vi "String to Parameter Type.vi"(0 "String in":string) -> (4 "Message Name":string, 6 "Parameters":T1[](array[typedef]), 8 "Parameter-1553":T1)   [LabVIEW 2011, in "AIT 1553 Custom Device.lvlib"]
uses:
  Controls/1553 Param.ctl
  AIT 1553 Custom Device.lvlib
panel:
  out "array":string[][](array[string])
  # "Message: Gun_One\nData_01,8,0,8,1.0000,0.0000,0\nMessage: Gun_Two\nData_02,8,0,8,1.0000,0.0000,0\nMessage: Get_It\nData_00,1,0,8,1.0000,0.0000,0"
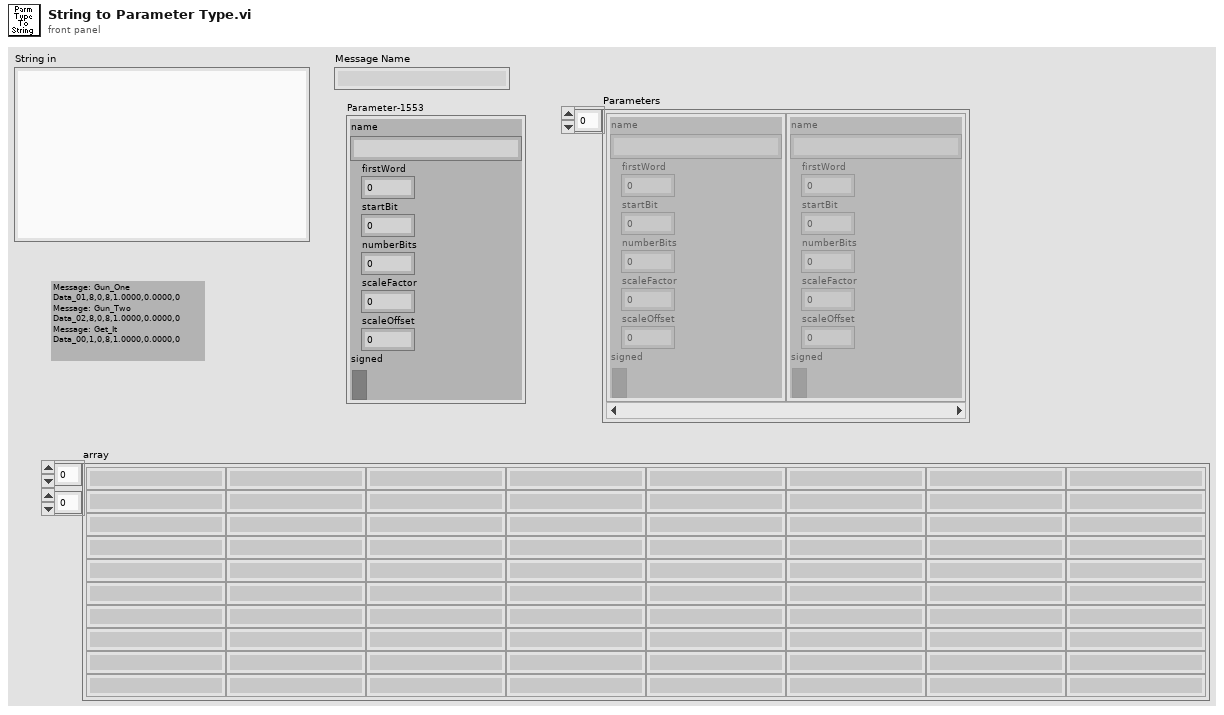
[diagram p1: front panel]
types:
  T1 = typedef "AIT 1553 Custom Device.lvlib/1553 Param.ctl" = cluster{"name":string, "firstWord":i32, "startBit":i32, "numberBits":i32, "scaleFactor":dbl, "scaleOffset":dbl, "signed":bool}
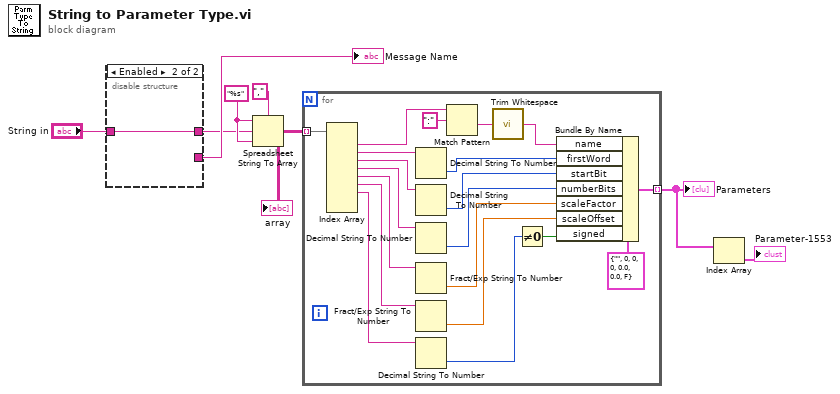
[diagram p0: block diagram]
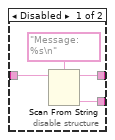
[diagram p2: hidden frame]
diagram:
  w5 = "%s" ("String")
  n1 = disable-structure shown="Enabled" {
    disable-tunnel: "String in" -> [w12 w13]
    disable-tunnel: [w10 _] -> w7
    disable-tunnel: [w9 w13] -> w4
    frame Disabled {
      n2 = Scan From String(format string="Message: %s\n", input string=w12) -> (remaining string=w9:string, output 1=w10:string)  [unwired: 3 in, 2 out]
    }
    frame Enabled {
    }
  }
  "Message Name" <- w7
  n3 = Spreadsheet String To Array(delimiter (Tab)=",", format string=w5, spreadsheet string=w4, array type (2D Dbl)=w5) -> (array=w3:string[][])
  "array" <- w3
  n4 = for {
    tunnel: [w31] -> w2 mode=indexing
    tunnel: w3 -> [w30] mode=indexing
    n5 = Index Array(array=w30) -> (element #1=w15:string, element #2=w29:string, element #3=w28:string, element #4=w27:string, element #5=w26:string, element #6=w25:string, element #7=w24:string)  [unwired: 9 in, 2 out]
    n6 = Decimal String To Number(string=w29) -> (number=w18:i32)  [unwired: 2 in, 1 out]
    n7 = Decimal String To Number(string=w28) -> (number=w19:i32)  [unwired: 2 in, 1 out]
    n8 = Decimal String To Number(string=w27) -> (number=w20:i32)  [unwired: 2 in, 1 out]
    n9 = Fract/Exp String To Number(string=w26) -> (number=w21:dbl)  [unwired: 3 in, 1 out]
    n10 = Fract/Exp String To Number(string=w25) -> (number=w22:dbl)  [unwired: 3 in, 1 out]
    n11 = Decimal String To Number(string=w24) -> (number=w23:i32)  [unwired: 2 in, 1 out]
    n12 = Match Pattern(string=w15, regular expression=":") -> (after substring=w16:string)  [unwired: 1 in, 3 out]
    n13 = call <vilib>:"Trim Whitespace.vi"("string"=w16) -> ("trimmed string"=w14:string)  [unwired: 1 in]
    n14 = Not Equal To 0?(x=w23) -> (x != 0?=w32:bool)
    n15 = Bundle By Name(cluster=T1 {"name"="", "firstWord"=0, "startBit"=0, "numberBits"=0, "scaleFactor"=0.0, "scaleOffset"=0.0, "signed"=FALSE} ("Parameter-1553"), "name"=w14, "firstWord"=w18, "startBit"=w19, "numberBits"=w20, "scaleFactor"=w21, "scaleOffset"=w22, "signed"=w32) -> (w31:T1)
  }
  "Parameters" <- w2
  n16 = Index Array(array=w2) -> (element=→"Parameter-1553":T1)  [unwired: 1 in]
